vi "Toggle.vi"(1 "Boolean":bool, 2 "Boolean 2":bool) -> (0 "Boolean 3":bool)   [LabVIEW 2017]
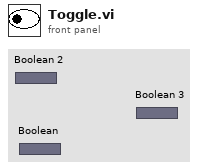
[diagram p1: front panel]
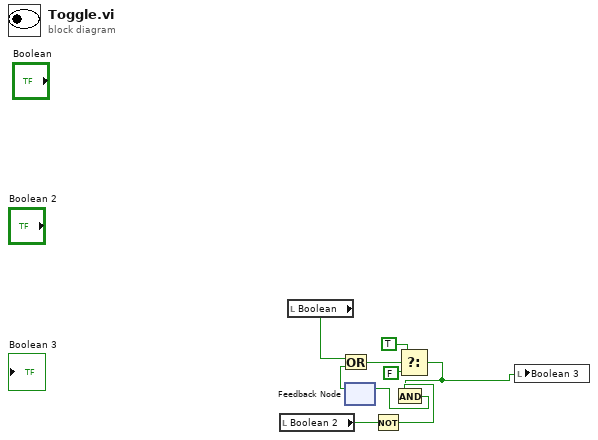
[diagram p0: block diagram]
diagram:
  n1 = local read "Boolean 2"() -> (w2:bool)
  n2 = local read "Boolean"() -> (w3:bool)
  n3 = feedback #1() -> (w4:bool)  [unwired: 1 in]
  n4 = Or(x=w3, y=w4) -> (x .or. y?=w7:bool)
  n5 = Not(x=w2) -> (.not. x?=w6:bool)
  n6 = Select(t=TRUE, s=w7, f=FALSE) -> (s? t:f=w1:bool)
  n7 = And(x=w1, y=w6) -> (x .and. y?=w5:bool)
  n8 = feedback-in #1(w5) -> ()
  n9 = local write "Boolean 3"(w1) -> ()
